vi "Item_OnPopupMenu.vi"(11 "Object":T1) -> ()   [LabVIEW 2020, in "Message Maker Provider.lvlib"]
uses:
  Message Maker Provider.lvlib
  <resource>/Framework/Providers/API/mxLvMenuItem.ctl
  Support/Localized Strings.vi
  AFPP Shared/Validation Mode.ctl
  AFPP Shared/AFPP Shared.lvlib
  <resource>/Framework/Providers/API/ItemRef.ctl
panel:
  out "error out":errorcluster
  in  "error in":errorcluster
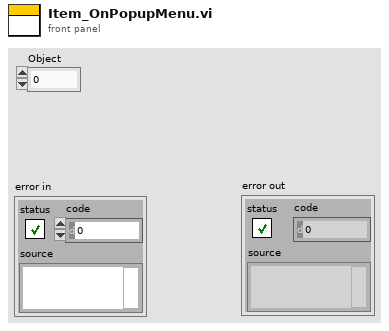
[diagram p1: front panel]
types:
  T1 = typedef "ItemRef.ctl" = u64
  T2 = typedef "AFPP Shared.lvlib/Validation Mode.ctl" = enum16{"An Actor Library", "A Target Tag"}
  T3 = typedef "mxLvMenuItem.ctl" = cluster{"Menu Name":string, "Description":string, "Icon File Name":path, "Menu Tag":string, "Enabled":bool, "Checked":bool, "Separator":bool, "Batchable":bool, "Weight":i32, "Batch Mode (Ignored if Not Batchable)":enum32{"Show If All Items Support Command", "Show If Any Items Support Command"}, "Menu Location":enum32{"<None>", "Project", "Project / Build Specifications", "Tools", "Tools / Source Control", "Tools / Real-Time Module", "Help"}, "Exclude From Getting Started Window Menu":bool}
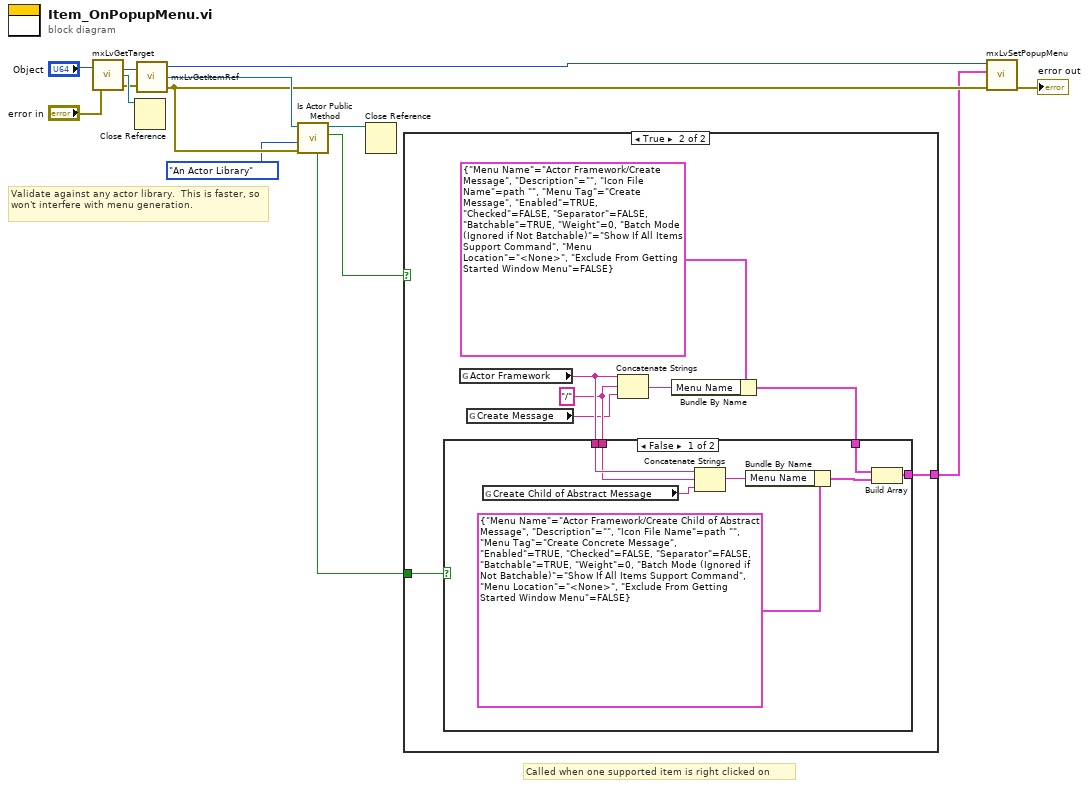
[diagram p0: block diagram]
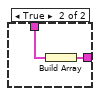
[diagram p3: hidden frame]
diagram:
  # "Validate against any actor library.  This is faster, so won't interfere with menu generation."
  # "Called when one supported item is right clicked on"
  n1 = call <resource>:"mxLvGetTarget.vi"("Item"="Object", "error in"="error in") -> ("Item"=w3:T1, "Target"=w7:refnum<vi>, "error out"=w6:errorcluster)
  n2 = Close Reference(reference=w7) -> ()  [unwired: 1 in, 1 out]
  n3 = call <resource>:"mxLvGetItemRef.vi"("Item"=w3, "error in"=w6) -> ("Item"=w10:T1, "Item Refnum"=w13:refnum<vi>, "error out"=w12:errorcluster)
  n4 = call "Is Actor Public Method.vi"("error in (no error)"=w12, "Validation"=Validation_Mode."An Actor Library", "ProjectItem in"=w13) -> ("Is Actor Public Method"=w8:bool, "ProjectItem out"=w14:refnum<vi>, "is actor interface?"=w1:bool)  [unwired: 5 in, 1 out]
  n5 = Close Reference(reference=w14) -> ()  [unwired: 1 in, 1 out]
  n6 = case shown="True" w8 {
    tunnel: [_ w20] -> w9
    tunnel: w1 -> [_ w15]
    frame False {
    }
    frame True {
      w17 = "/"
      n7 = global read "Localized Strings.vi" "Actor Framework"() -> (w18:string)
      n8 = global read "Localized Strings.vi" "Create Message"() -> (w16:string)
      n9 = Concatenate Strings(w18, w17, w16) -> (w19:string)
      n10 = Bundle By Name(cluster=T3 {"Menu Name"="Actor Framework/Create Message", "Description"="", "Icon File Name"=path "", "Menu Tag"="Create Message", "Enabled"=TRUE, "Checked"=FALSE, "Separator"=FALSE, "Batchable"=TRUE, "Weight"=0, "Batch Mode (Ignored if Not Batchable)"=enum."Show If All Items Support Command", "Menu Location"=enum."<None>", "Exclude From Getting Started Window Menu"=FALSE} ("Menu Item"), "Menu Name"=w19) -> (w21:T3)
      n11 = case shown="False" w15 {
        tunnel: w21 -> [w30 w32]
        tunnel: [w27 w31] -> w20
        tunnel: w18 -> [w25 _]
        tunnel: w17 -> [w24 _]
        frame False {
          n12 = global read "Localized Strings.vi" "Create Child of Abstract Message"() -> (w23:string)
          n13 = Concatenate Strings(w25, w24, w23) -> (w26:string)
          n14 = Bundle By Name(cluster=T3 {"Menu Name"="Actor Framework/Create Child of Abstract Message", "Description"="", "Icon File Name"=path "", "Menu Tag"="Create Concrete Message", "Enabled"=TRUE, "Checked"=FALSE, "Separator"=FALSE, "Batchable"=TRUE, "Weight"=0, "Batch Mode (Ignored if Not Batchable)"=enum."Show If All Items Support Command", "Menu Location"=enum."<None>", "Exclude From Getting Started Window Menu"=FALSE} ("Menu Item"), "Menu Name"=w26) -> (w28:T3)
          n15 = Build Array(w30, w28) -> (w27:T3[])
        }
        frame True {
          n16 = Build Array(w32) -> (w31:T3[])
        }
      }
    }
  }
  n17 = call <resource>:"mxLvSetPopupMenu.vi"("error in"=w12, "Popup Menu Items"=w9, "Item"=w10) -> ("error out"=→"error out":errorcluster)  [unwired: 7 in, 1 out]
